vi "HD_Device in Use.vi"   [LabVIEW 2016, in "General.lvlib"]
uses:
  General.lvlib
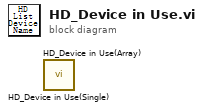
[diagram p0: block diagram]
diagram:
  n1 = call "HD_Device in Use(Single).vi"() -> ()  [unwired: 10 in, 2 out]
  n2 = call "HD_Device in Use(Array).vi"() -> ()  [unwired: 10 in, 2 out]
